vi "AddEventstoDB.vi"() -> ()   [LabVIEW 2014]
uses:
  <vilib>/addons/database/Connection.llb/DB Tools Open Connec (String).vi
  <vilib>/regexp/Match Regular Expression.xnode
  Backend/source/VI Source/FRCts20_Backend_Engine.lvlib
  <vilib>/addons/database/NI_Database_API.lvlib
panel:
  out "appended array":string[](array[string])
  # "Use this VI to read in the short event names file,\ncreate a Topic for each event, and add all this \ninformation to the database"
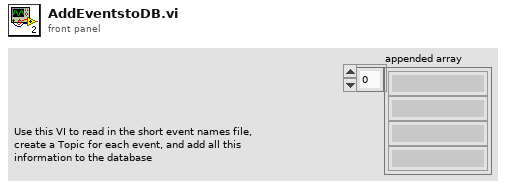
[diagram p1: front panel]
types:
  T1 = typedef "NI_Database_API.lvlib/Conn ObjectReference.ctl" = refnum<k1>
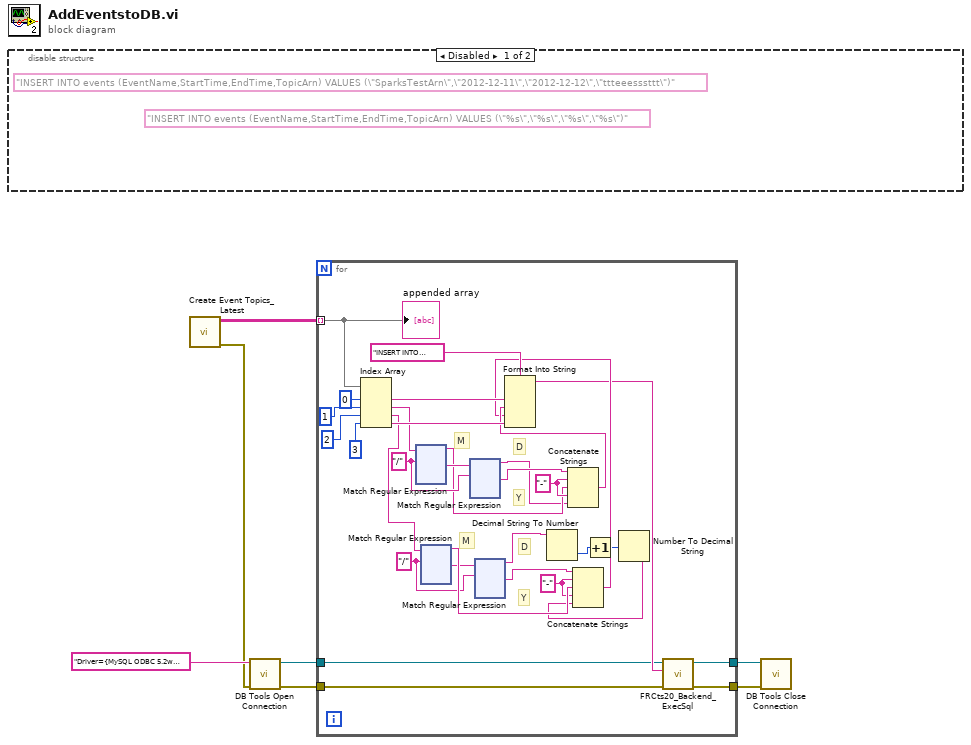
[diagram p0: block diagram]
diagram:
  n1 = disable-structure shown="Disabled" {
    frame Disabled {
      (unwired) "INSERT INTO events (EventName,StartTime,EndTime,TopicArn) VALUES (\"%s\",\"%s\",\"%s\",\"%s\")" ("format string")
      (unwired) "INSERT INTO events (EventName,StartTime,EndTime,TopicArn) VALUES (\"SparksTestArn\",\"2012-12-11\",\"2012-12-12\",\"ttteeesssttt\")" ("format string")
    }
    frame Enabled {
    }
  }
  n2 = call "Create Event Topics_Latest.vi"() -> ("error out"=w1:errorcluster, "appended array"=w2:string[][])  [unwired: 10 in]
  n3 = call-poly <vilib>:"DB Tools Open Connection.vi"("error in (no error)"=w1, "connection information"="Driver={MySQL ODBC 5.2w Driver};Server=parkway-production.cjlclmebggwl.us-east-1.rds.amazonaws.com;Database=parkway;User=parkway;Password=moonlightmarj" ("Connection String")) -> ("error out"=w5:errorcluster, "connection reference"=w6:T1)  [unwired: 6 in]
  n4 = for {
    tunnel: w2 -> [w37] mode=indexing
    tunnel: w6 -> [w13]
    tunnel: w5 -> [w16]
    tunnel: [w14] -> w3
    tunnel: [w13] -> w4
    w22 = "-" ("regular expression")
    w21 = "/" ("regular expression")
    w27 = "-" ("regular expression")
    w28 = "/" ("regular expression")
    # "Y"
    # "D"
    # "M"
    # "Y"
    # "D"
    # "M"
    n5 = Index Array(array=w37, index #1=0 ("index"), index #2=1 ("index"), index #3=2 ("index"), index #4=3 ("index")) -> (element #1=w32:string, element #2=w30:string, element #3=w19:string, element #4=w31:string)
    n6 = xnode "Match Regular Expression"("input string"=w30, "regular expression"=w28) -> ("before match"=w25:string, "after match"=w29:string)  [unwired: 4 in, 3 out]
    n7 = xnode "Match Regular Expression"("input string"=w19, "regular expression"=w21) -> ("before match"=w24:string, "after match"=w20:string)  [unwired: 4 in, 3 out]
    n8 = xnode "Match Regular Expression"("input string"=w29, "regular expression"=w28) -> ("before match"=w12:string, "after match"=w26:string)  [unwired: 4 in, 3 out]
    n9 = xnode "Match Regular Expression"("input string"=w20, "regular expression"=w21) -> ("before match"=w9:string, "after match"=w23:string)  [unwired: 4 in, 3 out]
    n10 = Decimal String To Number(string=w9) -> (number=w11:i32)  [unwired: 2 in, 1 out]
    n11 = Concatenate Strings(w26, w27, w25, w27, w12) -> (w18:string)
    n12 = Increment(x=w11) -> (x+1=w10:i32)
    n13 = Number To Decimal String(number=w10) -> (decimal integer string=w8:string)  [unwired: 1 in]
    n14 = Concatenate Strings(w23, w22, w24, w22, w8) -> (w17:string)
    n15 = Format Into String(format string="INSERT INTO events (EventName,StartTime,EndTime,TopicArn) VALUES (\"%s\",\"%s\",\"%s\",\"%s\")", w32, w18, w17, w31) -> (resulting string=w15:string)  [unwired: 2 in, 1 out]
    n16 = call "FRCts20_Backend_ExecSql.vi"("error in (no error)"=w16, "format string"=w15, "Refnum in"=w13) -> ("error out"=w14:errorcluster)  [unwired: 6 in, 2 out]
    "appended array" <- w37
  }
  n17 = call <vilib>:"DB Tools Close Connection.vi"("error in (no error)"=w3, "connection reference"=w4) -> ()  [unwired: 5 in, 1 out]
